vi "Get Formatted Function.vi"(8 "error in (no error)":errorcluster, 11 "Measure in":refnum<class "Measure.lvclass">) -> (0 "error out":errorcluster, 2 "Function":string, 3 "Measure out":refnum<class "Measure.lvclass">)   [LabVIEW 2023, in "HAF.lvlib" / "Measure.lvclass"]
doc: "Returns a Function name to insert into the command. If none has been configured then an empty string will be returned."
uses:
  Measure.lvclass
  Measure.lvclass/Measure.ctl
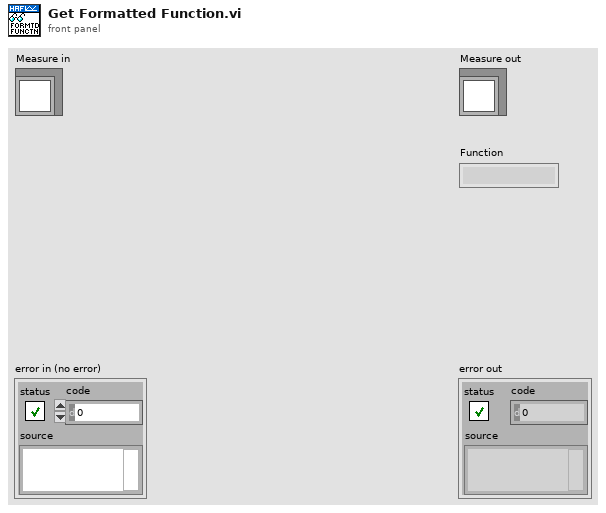
[diagram p1: front panel]
types:
  T1 = typedef "HAF.lvlib/Measure Function.ctl" = enum16{"[As Set]", "DC Voltage", "AC Voltage", "DC Current", "AC Current", "2-wire Resistance", "4-wire Resistance", "Diode", "Capacitance", "Temperature", "Continuity", "Frequency", "Period", "DC Voltage Ratio"}
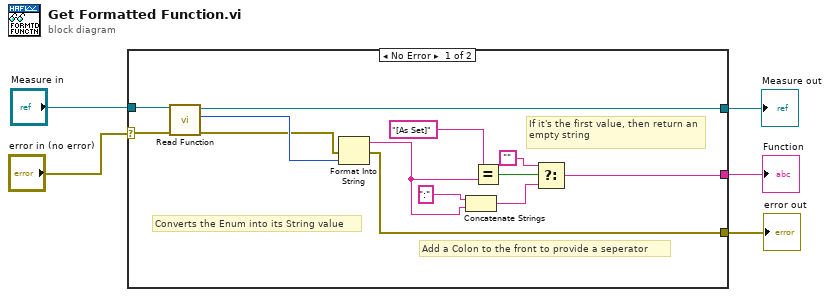
[diagram p0: block diagram]
diagram:
  n1 = case shown="No Error" "error in (no error)" {
    selector: "error in (no error)" -> [w17 w20]
    tunnel: [w13 w20] -> w4
    tunnel: [w16 w19] -> w2
    tunnel: "Measure in" -> [w18 w19]
    tunnel: [w10 _] -> w1
    frame No Error {
      # "Add a Colon to the front to provide a seperator"
      # "If it's the first value, then return an empty string"
      # "Converts the Enum into its String value"
      n2 = call-dynamic "Read Function.vi"("error in (no error)"=w17, "Measure in"=w18) -> ("error out"=w14:errorcluster, "Function"=w15:T1, "Measure out"=w16:refnum<class "Measure.lvclass">)  [unwired: 7 in]
      n3 = Format Into String(error in=w14, w15) -> (resulting string=w8:string, error out=w13:errorcluster)  [unwired: 2 in]
      n4 = Concatenate Strings(":" ("string"), w8) -> (w7:string)
      n5 = Equal?(x="[As Set]" ("y"), y=w8) -> (x = y?=w12:bool)
      n6 = Select(t="", s=w12, f=w7) -> (s? t:f=w10:string)
    }
    frame Error {
    }
  }
  "error out" <- w4
  "Measure out" <- w2
  "Function" <- w1
